vi "Parse.vi"(11 "address string":string) -> (3 "address":refnum<class "Generic Network Address.lvclass">)   [LabVIEW 2020, in "NI_WFCN.lvlib" / "Generic Network Address.lvclass"]
doc: "Parses a network address from the specified string. If parsing failed, returns a Generic Network Address initialized with the string, which will be considered invalid for future address manipulation."
uses:
  <vilib>/net/WFCN/Addressing/Generic Network Address/Generic Network Address.lvclass
  <vilib>/net/WFCN/Addressing/IPv4 Network Address/IPv4 Network Address.lvclass/IPv4 Network Address.ctl
  <vilib>/net/WFCN/Addressing/Generic Network Address/Generic Network Address.lvclass/Generic Network Address.ctl
  <vilib>/net/WFCN/Addressing/Hostname Network Address/Hostname Network Address.lvclass/Hostname Network Address.ctl
  <vilib>/net/WFCN/Utility/Is hostname mDNS.vi
  <vilib>/dlg_ctls.llb/Space Constant.vi
  <vilib>/net/WFCN/Addressing/IPv4 Network Address/IPv4 Network Address.lvclass
  e:/builds/penguin/labview/branches/2020/dev/dist/vi.lib/net/WFCN/Addressing/Generic Network Address/Generic Network Address.lvclass
  <vilib>/net/WFCN/Addressing/Hostname Network Address/Hostname Network Address.lvclass
  <vilib>/net/WFCN/Addressing/mDNS Hostname Network Address/mDNS Hostname Network Address.lvclass
  e:/builds/penguin/labview/branches/2020/dev/dist/vi.lib/net/WFCN/Addressing/Hostname Network Address/Hostname Network Address.lvclass
  <vilib>/Utility/error.llb/Error Cluster From Error Code.vi
  <vilib>/net/WFCN/NI_WFCN.lvlib
  <vilib>/net/WFCN/Addressing/MacOS Network Address/MacOS Network Address.lvclass
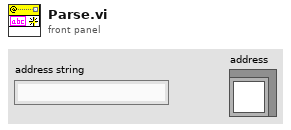
[diagram p1: front panel]
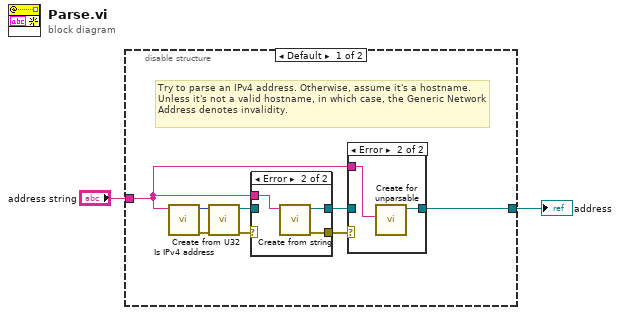
[diagram p0: block diagram]
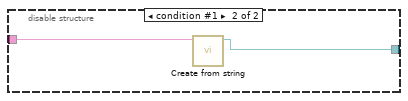
[diagram p4: hidden frame]
diagram:
  n1 = disable-structure shown="Default" {
    disable-tunnel: [w9 w18] -> w2
    disable-tunnel: "address string" -> [w8 w19]
    frame condition #0 (active) {
      # "Try to parse an IPv4 address. Otherwise, assume it's a hostname. Unless it's not a valid hostname, in which case, the Generic Network Address denotes invalidity."
      n2 = call <vilib>:"Is IPv4 address.vi"("address string"=w8) -> ("error out"=w5:errorcluster, "address U32"=w6:u32)  [unwired: 9 in]
      n3 = call <vilib>:"Create from U32.vi"("address U32"=w6) -> ("address out"=w4:refnum<class "IPv4 Network Address.lvclass">)  [unwired: 10 in]
      n4 = case shown="Error" w5 {
        selector: w5 -> [w13 _]
        tunnel: w4 -> [w14 _]
        tunnel: [w14 w16] -> w7
        tunnel: [w13 w15] -> w3
        tunnel: w8 -> [_ w17]
        frame No Error {
        }
        frame Error {
          n5 = call <vilib>:"Create from string.vi"("address"=w17) -> ("error out"=w15:errorcluster, "Hostname Network Address out"=w16:refnum<class "Generic Network Address.lvclass">)  [unwired: 9 in]
        }
      }
      n6 = case shown="Error" w3 {
        tunnel: w7 -> [w10 _]
        tunnel: [w10 w11] -> w9
        tunnel: w8 -> [_ w12]
        frame No Error {
        }
        frame Error {
          n7 = call <vilib>:"Create for unparsable.vi"("hostname"=w12) -> ("Generic Network Address out"=w11:refnum<class "Generic Network Address.lvclass">)  [unwired: 10 in]
        }
      }
    }
    frame condition #1 {
      n8 = call <vilib>:"Create from string.vi"("address string"=w19) -> ("address"=w18:refnum<class "MacOS Network Address.lvclass">)  [unwired: 10 in]
    }
  }
  "address" <- w2
